vi "Set Timer Enabled.vi"(8 "error in (no error)":errorcluster, 10 "Timer Config":T1={"Name"="", "Period [s]"=0.0, "Enabled"=TRUE, "Metadata"=""}, 11 "Timers Manager Actor in":refnum<class "Task Scheduler Actor.lvclass">) -> (0 "error out":errorcluster, 3 "Timers Manager Actor out":refnum<class "Task Scheduler Actor.lvclass">)   [LabVIEW 2015, in "Task Scheduler Actor.lvclass"]
uses:
  Task Scheduler Actor.lvclass
  Timer Config.ctl
  Task Scheduler Actor.lvclass/Task Scheduler Actor.ctl
  Re-use Libraries/Timer/Timer.lvclass/Timer.ctl
  Re-use Libraries/Timer/Timer.lvclass
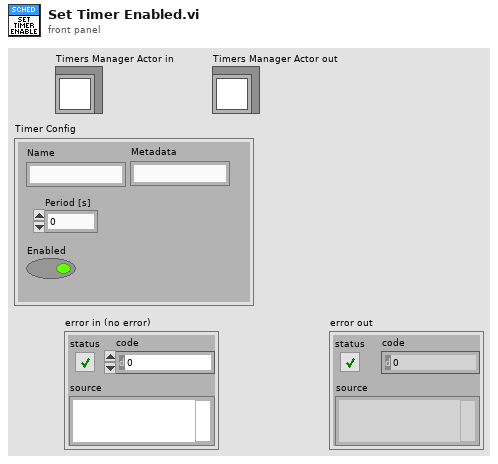
[diagram p1: front panel]
types:
  T1 = typedef "Task Scheduler Actor.lvclass/Timer Config.ctl" = cluster{"Name":string, "Period [s]":dbl, "Enabled":bool, "Metadata":string}
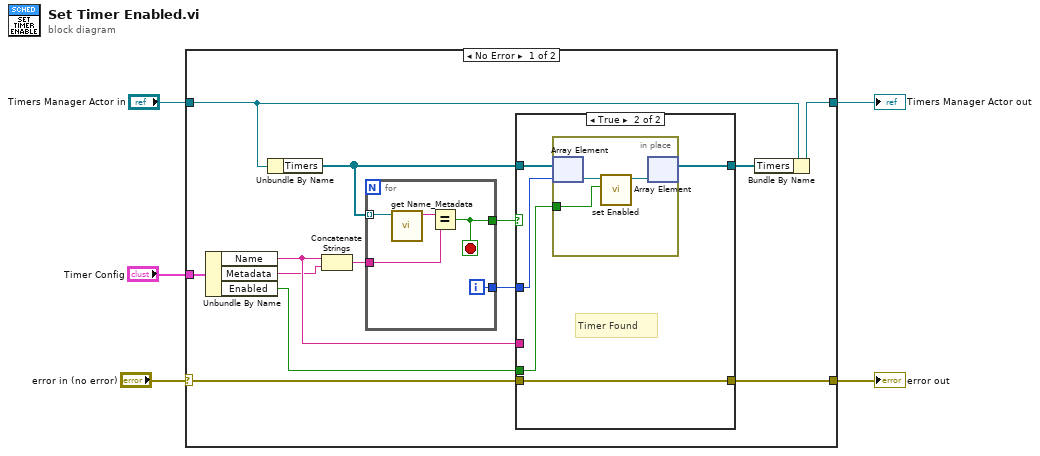
[diagram p0: block diagram]
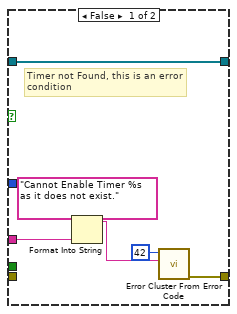
[diagram p2: hidden frame]
diagram:
  n1 = case shown="No Error" "error in (no error)" {
    selector: "error in (no error)" -> [w12 w39]
    tunnel: [w17 w38] -> w5
    tunnel: "Timers Manager Actor in" -> [w16 w38]
    tunnel: "Timer Config" -> [w11 _]
    tunnel: [w13 w39] -> w2
    frame No Error {
      n2 = Unbundle By Name(w11) -> ("Name"=w8:string, "Metadata"=w7:string, "Enabled"=w10:bool)
      n3 = Unbundle By Name(w16) -> ("Timers"=w15:refnum<class "Timer.lvclass">[])
      n4 = Concatenate Strings(w8, w7) -> (w6:string)
      n5 = for {
        tunnel: w15 -> [w37] mode=indexing
        tunnel: [w35] -> w9
        tunnel: [w34] -> w14
        tunnel: w6 -> [w33]
        i -> [w35]
        stop <- w34 stop-if-true
        n6 = call "get Name_Metadata .vi"("Timer in"=w37) -> ("Name"=w36:string)  [unwired: 10 in]
        n7 = Equal?(x=w36, y=w33) -> (x = y?=w34:bool)
      }
      n8 = case shown="True" w14 {
        tunnel: w8 -> [w20 _]
        tunnel: w15 -> [w24 w28]
        tunnel: [w24 w26] -> w18
        tunnel: [w23 w29] -> w13
        tunnel: w12 -> [_ w29]
        tunnel: w10 -> [_ w25]
        tunnel: w9 -> [_ w27]
        frame False {
          # "Timer not Found, this is an error condition"
          n9 = Format Into String(format string="Cannot Enable Timer %s as it does not exist.", w20) -> (resulting string=w19:string)  [unwired: 2 in, 1 out]
          n10 = call <vilib>:"Error Cluster From Error Code.vi"("error message (\"\")"=w19, "error code (0)"=42) -> ("error out"=w23:errorcluster)  [unwired: 7 in]
        }
        frame True {
          # "Timer Found"
          n11 = in-place {
            in-place-border: w25 -> [w30]
            n12 = in-place-array #1(w28, w27) -> (w32:refnum<class "Timer.lvclass">)
            n13 = call "set Enabled.vi"("Enabled"=w30, "Timer in"=w32) -> ("Timer out"=w31:refnum<class "Timer.lvclass">)  [unwired: 9 in]
            n14 = in-place-array #1(w31) -> (w26:refnum<class "Timer.lvclass">[])  [unwired: 1 out]
          }
        }
      }
      n15 = Bundle By Name(cluster=w16, "Timers"=w18) -> (w17:refnum<class "Task Scheduler Actor.lvclass">)
    }
    frame Error {
    }
  }
  "Timers Manager Actor out" <- w5
  "error out" <- w2
